vi "Teleop.vi"(10 "Match Info":T1={"Autonomous Elapsed Seconds"=0.0, "TeleOp Elapsed Seconds"=0.0, "Disabled Elapsed Seconds"=0.0, "Visited Autonomous"=FALSE, "Visited TeleOp"=FALSE, "Visited Disabled"=FALSE, "Autonomous Settings"={"Autonomous Style"=enum."Independent", "VI Refnum"=refnum}}, 11 "Call Context":T2) -> ()   [LabVIEW 2023]
doc: "This VI is called for each enabled TeleOp packet received from the DS. It is typically used to read from joysticks and other inputs and update I/O or setpoints for timed control loops. It should complete and return within 20 milliseconds or risk missing DS packets."
uses:
  <vilib>/Rock Robotics/WPI/DriverStation/WPI_DriverStationDerivedRobotMode.ctl
  <vilib>/Rock Robotics/WPI/DriverStation/WPI_DriverStationMatch Info.ctl
  <vilib>/Rock Robotics/WPI/Joystick/XBox Buttons Indexer.ctl
  <vilib>/Rock Robotics/WPI/Joystick/XBox Axes Indexer.ctl
  Swerve/Implementation/Swerve Setpoints2.ctl
  Swerve/Implementation/Swerve Operations.ctl
  <vilib>/Rock Robotics/WPI/Utilities/WPI_GetSetVariantRefNum.vi
  <vilib>/Rock Robotics/Network Tables/NT Write Boolean Array.vi
  <vilib>/Rock Robotics/Network Tables/NT Write Numeric Array.vi
  <vilib>/Rock Robotics/Network Tables/NT Read Float.vi
  Framework/Robot Global Data.vi
  <vilib>/Rock Robotics/Network Tables/NT Read Boolean.vi
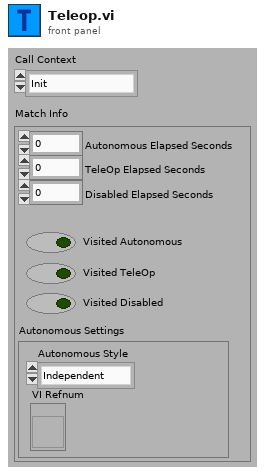
[diagram p1: front panel]
types:
  T1 = typedef "WPI_DriverStationMatch Info.ctl" = cluster{"Autonomous Elapsed Seconds":dbl, "TeleOp Elapsed Seconds":dbl, "Disabled Elapsed Seconds":dbl, "Visited Autonomous":bool, "Visited TeleOp":bool, "Visited Disabled":bool, "Autonomous Settings":cluster{"Autonomous Style":enum16{"Iterative", "Independent"}, "VI Refnum":refnum<vi>}}
  T2 = typedef "WPI_DriverStationDerivedRobotMode.ctl" = enum16{"Init", "Execute", "Stop"}
  T3 = typedef "XBox Axes Indexer.ctl" = enum16{"Left X", "Left Y", "Left Trigger", "Right Trigger", "Right X", "Right Y"}
  T4 = typedef "XBox Buttons Indexer.ctl" = enum16{"A", "B", "X", "Y", "Left Bumper", "Right Bumper", "Back", "Start", "Left Joystick", "Right Joystick"}
  T5 = typedef "WPI_JoystickDevRef.ctl" = cluster{"Device":T6}
  T6 = typedef "WPI_JoystickDeviceEnum.ctl" = enum16{"USB 0", "USB 1", "USB 2", "USB 3", "USB 4", "USB 5"}
  T7 = typedef "ADIS16470 Device Reference.ctl" = cluster{"DevStatus":errorcluster, "Hardware Config":T8, "Calibration Complete":refnum<notifier>, "Status Reference":refnum<data-value>, "Data Reference":refnum<data-value>, "Sychronous Process VI":T12, "Cmd FIFO":refnum<k33>, "Source":T13, "Data FIFO":refnum<k33>, "Calibration Time (ms)":u32, "Data Reference":refnum<data-value>}
  T8 = typedef "ADIS16470 Hardware Configuration.ctl" = cluster{"SPI Clock Rate (Hz)":dbl, "IMU SPI Mode (3)":T9, "IMU Reset Pin":T10, "IMU SPI Bus":T11, "IMU Data Ready Pin":T10, "Stall Config":cluster{"Pow2BytesPerRead":u8, "StallTicks":u16, "CsToSclkTicks":u8}}
  T9 = typedef "WPI_SPIMode.ctl" = enum16{"Mode 0 (Clk Idle Low,Sample on Leading)", "Mode 1 (Clk Idle Low,Sample on Trailing)", "Mode 2 (Clk Idle High,Sample on Leading)", "Mode 3 (Clk Idle High,Sample on Trailing)"}
  T10 = typedef "FPGA_DIOChannel.ctl" = enum8{"DIO 0", "DIO 1", "DIO 2", "DIO 3", "DIO 4", "DIO 5", "DIO 6", "DIO 7", "DIO 8", "DIO 9", "DIO MXP 0", "DIO MXP 1", "DIO MXP 2", "DIO MXP 3", "DIO MXP 4", "DIO MXP 5", "DIO MXP 6", "DIO MXP 7", "DIO MXP 8", "DIO MXP 9", "DIO MXP 10", "DIO MXP 11", "DIO MXP 12", "DIO MXP 13", "DIO MXP 14", "DIO MXP 15", "SPI Port CS1", "SPI Port CS2", "SPI Port CS3", "SPI Port MISO", "SPI Port MOSI", "Invalid"}
  T11 = typedef "spi_bus.ctl" = enum16{"SPI On-Board, CS0", "SPI On-Board, CS1", "SPI On-Board, CS2", "SPI On-Board, CS3", "SPI MXP", "Invalid"}
  T12 = typedef "ADIS16470 Process.ctl" = refnum<vi>
  T13 = typedef "FPGA_CounterEncoderSourceConvertionLVSourceType.ctl" = cluster{"DevStatus":errorcluster, "AnalogTriggerMode?":bool, "DigitalMode":cluster{"DIO Channel":T14}, "AnalogTriggerMode":cluster{"AnalogTriggerIndex":T15, "OutputType":T16}}
  T14 = typedef "FPGA_DIODigitalSourceChannel.ctl" = enum8{"DIO 0", "DIO 1", "DIO 2", "DIO 3", "DIO 4", "DIO 5", "DIO 6", "DIO 7", "DIO 8", "DIO 9", "DIO MXP 0", "DIO MXP 1", "DIO MXP 2", "DIO MXP 3", "DIO MXP 4", "DIO MXP 5", "DIO MXP 6", "DIO MXP 7", "DIO MXP 8", "DIO MXP 9", "DIO MXP 10", "DIO MXP 11", "DIO MXP 12", "DIO MXP 13", "DIO MXP 14", "DIO MXP 15", "SPI Port CS1", "SPI Port CS2", "SPI Port CS3", "SPI Port MISO", "SPI Port MOSI", "Disabled"}
  T15 = typedef "FPGA_AnalogTriggerIndex.ctl" = enum8{"Trig 0", "Trig 1", "Trig 2", "Trig 3", "Trig 4", "Trig 5", "Trig 6", "Trig 7", "Invalid"}
  T16 = typedef "FPGA_AnalogTriggerOutType.ctl" = enum16{"InWindow", "TriggerState", "Rising", "Falling"}
  T17 = typedef "ADIS16470 Data.ctl" = cluster{"XAngle":dbl, "YAngle":dbl, "ZAngle":dbl}
  T18 = typedef "Swerve Setpoints2.ctl" = cluster{"Operation":T19, "Gyro":dbl, "FWD":dbl, "STR":dbl, "X rotate":dbl, "Y rotate":dbl, "Time":dbl, "Distance":dbl, "Right Trigger":dbl, "Angle":dbl, "Start Angle":dbl, "Tag ID":dbl, "Start Positions":dbl[]}
  T19 = typedef "Swerve Operations.ctl" = enum16{"Reserve", "Read Current", "Immediate", "Stop", "Balance", "Direct  Joystick Drive", "Joystick Drive", "Drive for Distance", "Drive for Time", "Turn to Angle", "Drive to Angle(Time)", "Drive to Angle(Distance)", "Look At Cone", "Look At Cube", "Move To Tape", "Move To Tag"}
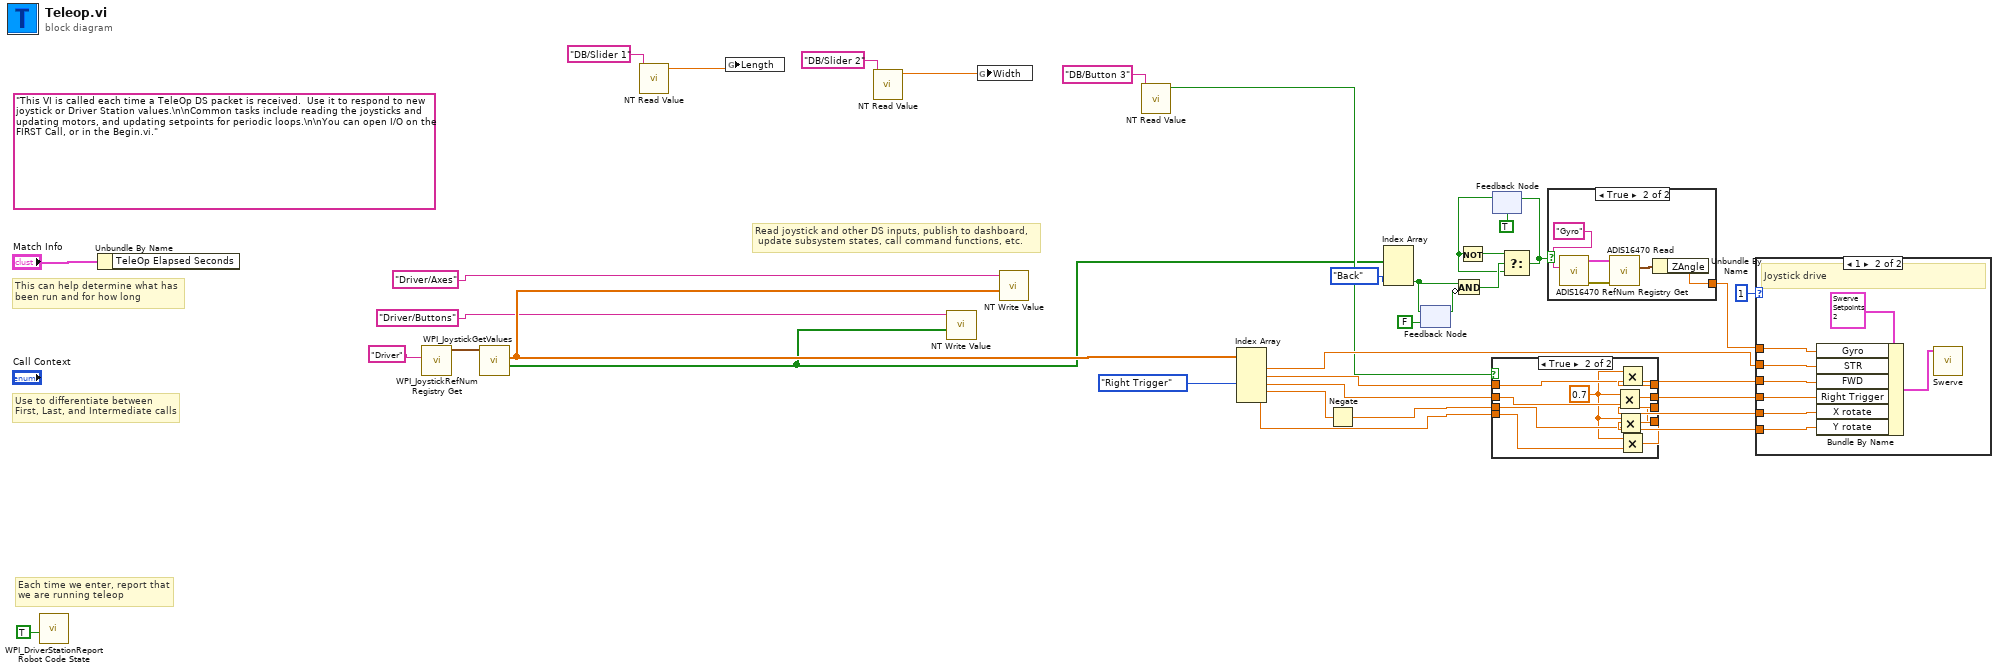
[diagram p0: block diagram]
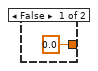
[diagram p2: hidden frame]
diagram:
  (unwired) "This VI is called each time a TeleOp DS packet is received.  Use it to respond to new joystick or Driver Station values.\n\nCommon tasks include reading the joysticks and updating motors, and updating setpoints for periodic loops.\n\nYou can open I/O on the FIRST Call, or in the Begin.vi."
  # "Read joystick and other DS inputs, publish to dashboard,\n update subsystem states, call command functions, etc."
  # "Each time we enter, report that\nwe are running teleop"
  # "Use to differentiate between\nFirst, Last, and Intermediate calls"
  # "This can help determine what has\nbeen run and for how long"
  n1 = call <vilib>:"WPI_DriverStationReport Robot Code State.vi"("TeleOp"=TRUE ("Autonomous")) -> ()  [unwired: 10 in, 1 out]
  n2 = Unbundle By Name("Match Info") -> ()  [unwired: 1 out]
  n3 = call <vilib>:"WPI_JoystickRefNum Registry Get.vi"("refnum name"="Driver") -> ("JoystickDevRef"=w33:T5)  [unwired: 1 in, 9 out]
  n4 = call <vilib>:"WPI_JoystickGetValues.vi"("JoystickDevRef"=w33) -> ("Buttons"=w13:bool[], "Axes"=w32:dbl[])  [unwired: 6 in, 3 out]
  n5 = call-poly <vilib>:"NT Read Value.vi"("name"="DB/Slider 1") -> ("value"=w26:dbl)  [unwired: 8 in, 2 out]
  n6 = global write "Robot Global Data.vi" "Length"(w26) -> ()
  n7 = call-poly <vilib>:"NT Read Value.vi"("name"="DB/Slider 2") -> ("value"=w24:dbl)  [unwired: 8 in, 2 out]
  n8 = call-poly <vilib>:"NT Write Value.vi"("value"=w13, "name"="Driver/Buttons" ("Name")) -> ()  [unwired: 9 in, 1 out]
  n9 = global write "Robot Global Data.vi" "Width"(w24) -> ()
  n10 = call-poly <vilib>:"NT Write Value.vi"("value"=w32, "name"="Driver/Axes" ("Name")) -> ()  [unwired: 9 in, 1 out]
  n11 = call-poly <vilib>:"NT Read Value.vi"("name"="DB/Button 3") -> ("value"=w22:bool)  [unwired: 8 in, 2 out]
  n12 = Index Array(array=w32, index #3=XBox_Axes_Indexer."Right Trigger" ("XBox Axes")) -> (element #1=w28:dbl, element #2=w21:dbl, element #3=w19:dbl, element #4=w2:dbl, element #5=w15:dbl)  [unwired: 4 in]
  n13 = Negate(x=w2) -> (-x=w17:dbl)
  n14 = Index Array(array=w13, index #3=XBox_Buttons_Indexer."Back" ("XBox Buttons")) -> (element #3=w11:bool)  [unwired: 2 in, 2 out]
  n15 = feedback-in #1(w11) -> ()
  n16 = feedback #1(FALSE) -> (w10:bool)
  n17 = Compound Arithmetic op=AND(w11, invert w10) -> (w9:bool)
  n18 = case shown="True" w22 {
    tunnel: w21 -> [w40 w49]
    tunnel: [w40 w45] -> w20
    tunnel: w19 -> [w39 w48]
    tunnel: [w39 w44] -> w18
    tunnel: w17 -> [w38 w47]
    tunnel: [w38 w43] -> w16
    tunnel: w15 -> [w37 w46]
    tunnel: [w37 w42] -> w14
    frame False {
    }
    frame True {
      w41 = 0.7 ("x")
      n19 = Multiply(x=w41, y=w48) -> (x*y=w44:dbl)
      n20 = Multiply(x=w41, y=w47) -> (x*y=w43:dbl)
      n21 = Multiply(x=w41, y=w49) -> (x*y=w45:dbl)
      n22 = Multiply(x=w41, y=w46) -> (x*y=w42:dbl)
    }
  }
  n23 = feedback #2(TRUE) -> (w7:bool)
  n24 = Not(x=w7) -> (.not. x?=w8:bool)
  n25 = Select(t=w8, s=w9, f=w7) -> (s? t:f=w6:bool)
  n26 = feedback-in #2(w6) -> ()
  n27 = case shown="True" w6 {
    tunnel: [0.0 ("ZAngle") w55] -> w29
    frame False {
    }
    frame True {
      n28 = call <vilib>:"ADIS16470 RefNum Registry Get.vi"("refnum name"="Gyro") -> ("error out"=w52:errorcluster, "ADIS16470DevRef out"=w53:T7)  [unwired: 9 in]
      n29 = call <vilib>:"ADIS16470 Read.vi"("error in (no error)"=w52, "ADIS16470DevRef"=w53) -> ("ADIS16470 Value"=w54:T17)  [unwired: 6 in, 3 out]
      n30 = Unbundle By Name(w54) -> ("ZAngle"=w55:dbl)
    }
  }
  n31 = case shown="1" 1 {
    tunnel: w29 -> [_ w61]
    tunnel: w18 -> [_ w60]
    tunnel: w16 -> [_ w59]
    tunnel: w20 -> [_ w58]
    tunnel: w28 -> [_ w57]
    tunnel: w14 -> [_ w56]
    frame 0, Default {
    }
    frame 1 {
      # "Joystick drive"
      n32 = Bundle By Name(cluster=T18 {"Operation"=enum."Joystick Drive", "Gyro"=0.0, "FWD"=0.0, "STR"=0.0, "X rotate"=0.0, "Y rotate"=0.0, "Time"=0.0, "Distance"=0.0, "Right Trigger"=0.0, "Angle"=0.0, "Start Angle"=0.0, "Tag ID"=0.0, "Start Positions"=[]} ("SubSystem Data"), "Gyro"=w61, "STR"=w57, "FWD"=w58, "Right Trigger"=w60, "X rotate"=w59, "Y rotate"=w56) -> (w62:T18)
      n33 = call "Swerve.vi"("SubSystem Data"=w62) -> ()  [unwired: 10 in, 1 out]
    }
  }
